vi "Subvi DO.vi"(8 "DO in":bool, 9 "Nmax":u32, 10 "Memory label":refnum<k21>, 11 "DO channel":refnum<k21>) -> (0 "DO out":bool)   [LabVIEW 2017]
uses:
  <vilib>/rvi/Emulation/niFpgaGetClockAttributes.vi
  <vilib>/rvi/Emulation/niFpgaSctlEmulationGetInTimedLoop.vi
  <vilib>/rvi/Emulation/niFpgaEmulationReportErrorSimple.vi
  GV DO delay.vi
  <vilib>/rvi/eio/common/nirviEmuTemplateMethod_errors.vi
  <vilib>/rvi/DataTransferAndStorage/Container/Common/niFpgaContainerExecOnDevCompGetState.vi
  <vilib>/rvi/Emulation/niFpgaEmulationIsFPGAContextNoSignature.vi
  <vilib>/rvi/DataTransferAndStorage/Container/Common/niFpgaContainerGetUniqueNameForEmu.vi
  <vilib>/rvi/Emulation/niFpgaProcessEmulError.vi
  <vilib>/rvi/errors/nirviReportUnexpectedCaseInternalError (U32).vi
  <vilib>/rvi/Memory/Memory_Emulation/niFpgaMemoryEmulationCacheClearOnFirstRun.vi
  <vilib>/rvi/Memory/Memory_Emulation/nirvimemoryEmulationManagerCache_MakeExclusive.vi
  <vilib>/rvi/Memory/Memory_Emulation/niFpgaMemoryEmulationValidateCache.vi
  <vilib>/rvi/Memory/Memory_Emulation/nirvimemoryEmulationManagerCache_InsertValue.vi
  <vilib>/Utility/error.llb/Clear Errors.vi
  <vilib>/rvi/Memory/Memory_Emulation/nirvimemoryEmulationManagerCache_ReleaseExclusive.vi
  <vilib>/rvi/Memory/Memory_Emulation/nirvimemoryEmulationManagerCache_GetValue.vi
  <vilib>/rvi/Memory/Memory_Emulation/nirvimemoryEmulationManagerCache_SetValue.vi
  <vilib>/rvi/Emulation/niFpgaSctlEmulationResourceMgr.vi
  <vilib>/rvi/Emulation/niFpgaCriticalErrorInLSC.vi
  GV trigger.vi
  <vilib>/eio/EIONode/EIONode.xnode
  <vilib>/rvi/DataTransferAndStorage/Container/XNode/niFpgaContainer.xnode
  <vilib>/rvi/Memory/Memory_Emulation/niFpgaMemoryEmulationRefIn.vi
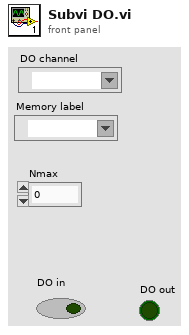
[diagram p1: front panel]
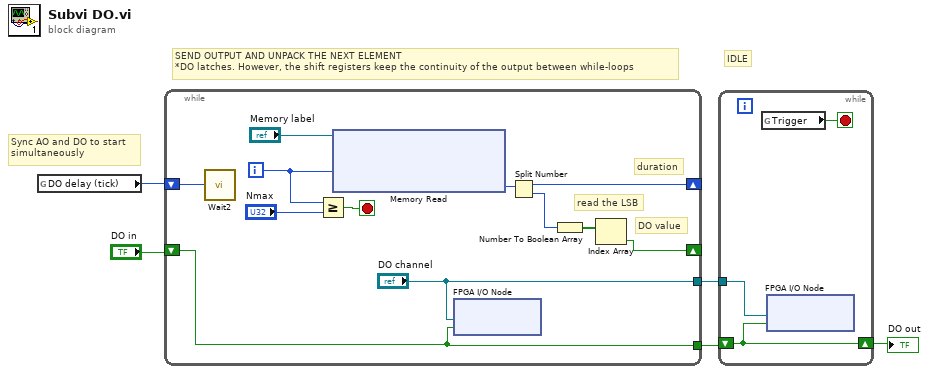
[diagram p0: block diagram]
diagram:
  # "IDLE"
  # "SEND OUTPUT AND UNPACK THE NEXT ELEMENT\n*DO latches. However, the shift registers keep the continuity of the output between while-loops"
  # "Sync AO and DO to start\nsimultaneously"
  n1 = global read "GV DO delay.vi" "DO delay (tick)"() -> (w5:u16)
  n2 = while {
    shift-right: [w9] -> _
    shift-left: "DO in" -> [w6]
    tunnel: [w6] -> w3
    shift-right: [w12] -> _
    shift-left: w5 -> [w11]
    tunnel: ["DO channel"] -> w1
    i -> [w8]
    stop <- w7 stop-if-true
    # "read the LSB"
    # "DO value"
    # "duration"
    n3 = call "Wait2"("Count(Ticks)"=w11) -> ()  [unwired: 1 out]
    n4 = Greater Or Equal?(x=w8, y="Nmax") -> (x >= y?=w7:bool)
    n5 = xnode ("Memory Read")("Address"=w8, "Memory In"="Memory label") -> ("Data"=w16:u32)  [unwired: 1 out]
    n6 = xnode "FPGA I/O Node"("I/O Item"=w6, "FPGA I/O In"="DO channel") -> ()  [unwired: 1 out]
    n7 = Split Number(x=w16) -> (hi(x)=w12:u16, lo(x)=w13:u16)
    n8 = Number To Boolean Array(number=w13) -> (Boolean array=w17:bool[])
    n9 = Index Array(array=w17) -> (element=w9:bool)  [unwired: 1 in]
  }
  n10 = while {
    shift-right: [w19] -> w2
    shift-left: w3 -> [w19]
    tunnel: w1 -> [w20]
    stop <- w18 stop-if-true
    n11 = global read "GV trigger.vi" "Trigger"() -> (w18:bool)
    n12 = xnode "FPGA I/O Node"("I/O Item"=w19, "FPGA I/O In"=w20) -> ()  [unwired: 1 out]
  }
  "DO out" <- w2
